vi "SerialServer.vi"(5 "Stop Refnum":refnum<vi>, 6 "Local Port":u16=16505) -> (0 "error out":errorcluster, 3 "FPGA VI Reference Out":refnum<k20>)   [LabVIEW 2013]
panel:
  out "Baud Rate":i32(ring)=1 items=["9600"=1, "19200"=2, "38400"=4, "57600"=8, "115200"=16, "230400"=32, "460800"=64, "921600"=128]
  out "OverRunError":bool
  in  "Flush on Close":bool
  out "UART TX count":u64
  out "UART RX count":u64
  out "TCP Bytes Out":u64
  out "Elements in UART TX Queue":i32
  out "Elements in UART RX Queue":i32
  out "TCP Bytes In":u64
  out "connection ID":refnum<k5>
  out "Connected?":bool
  out "Stopped?":bool caption="BeenStopped?"
  out "Remote Address":string
  out "Remote Port":u16
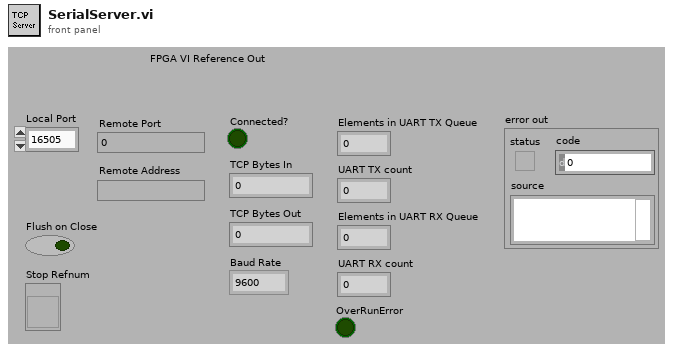
[diagram p1: front panel]
types:
  T1 = typedef "FPGA_Reference.ctl" = refnum<k20>
  T2 = enum16{"Standard", "Buffered", "CRLF", "Immediate"}
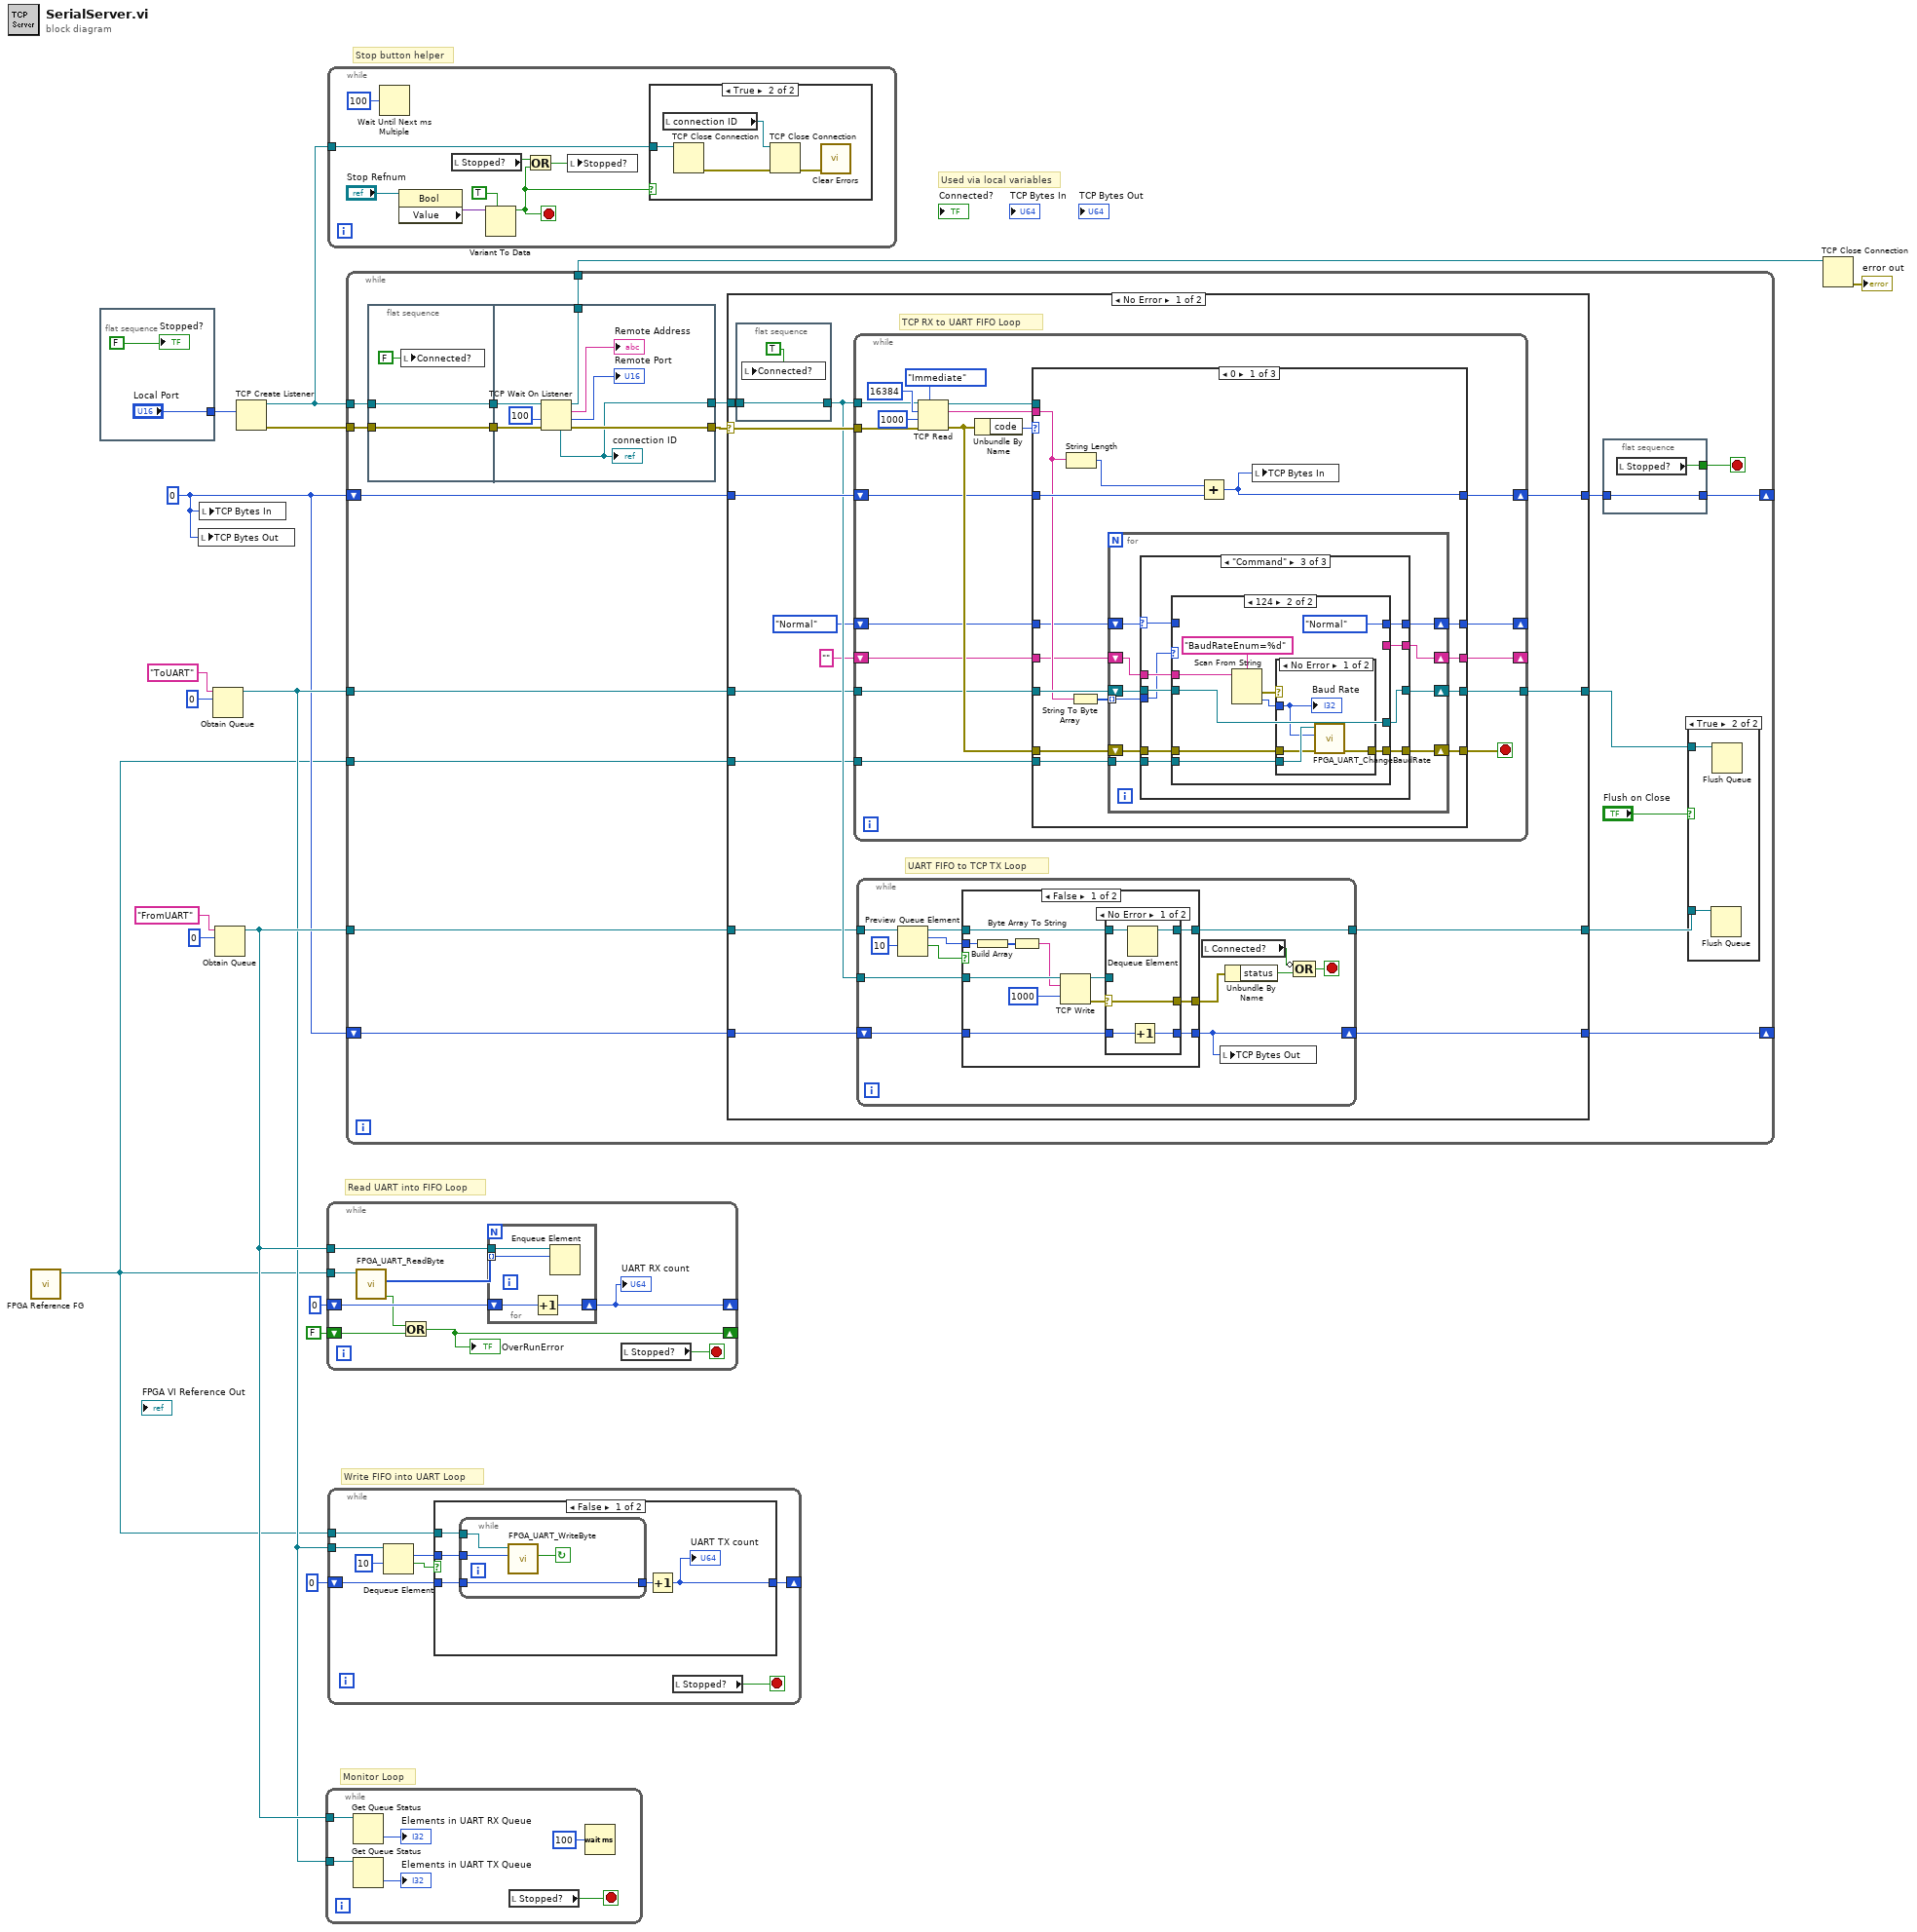
[diagram p0: block diagram]
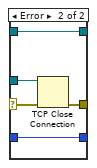
[diagram p5: hidden frame]
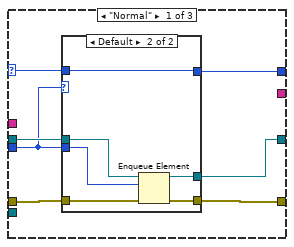
[diagram p7: hidden frame]
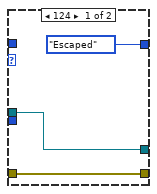
[diagram p8: hidden frame]
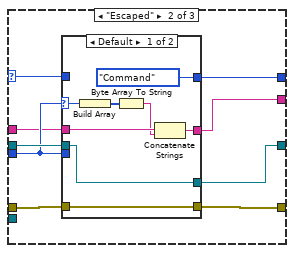
[diagram p9: hidden frame]
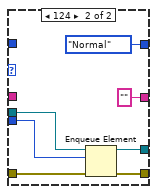
[diagram p10: hidden frame]
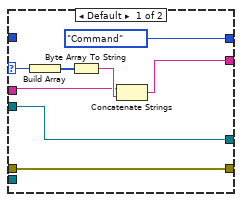
[diagram p11: hidden frame]
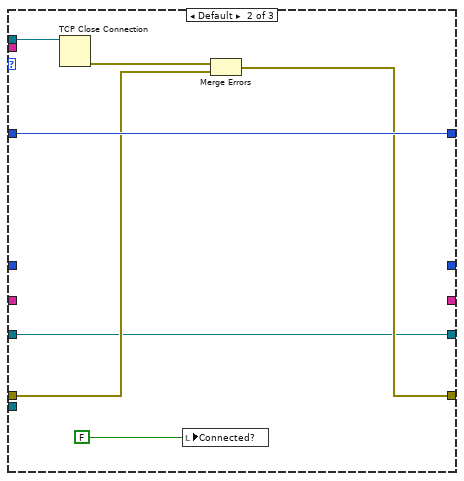
[diagram p13: hidden frame]
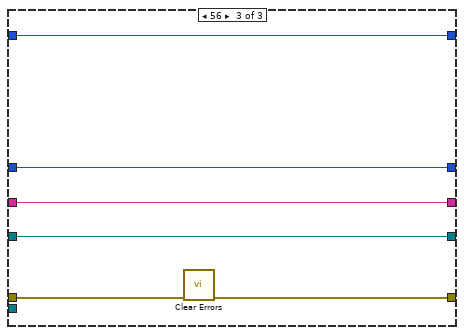
[diagram p14: hidden frame]
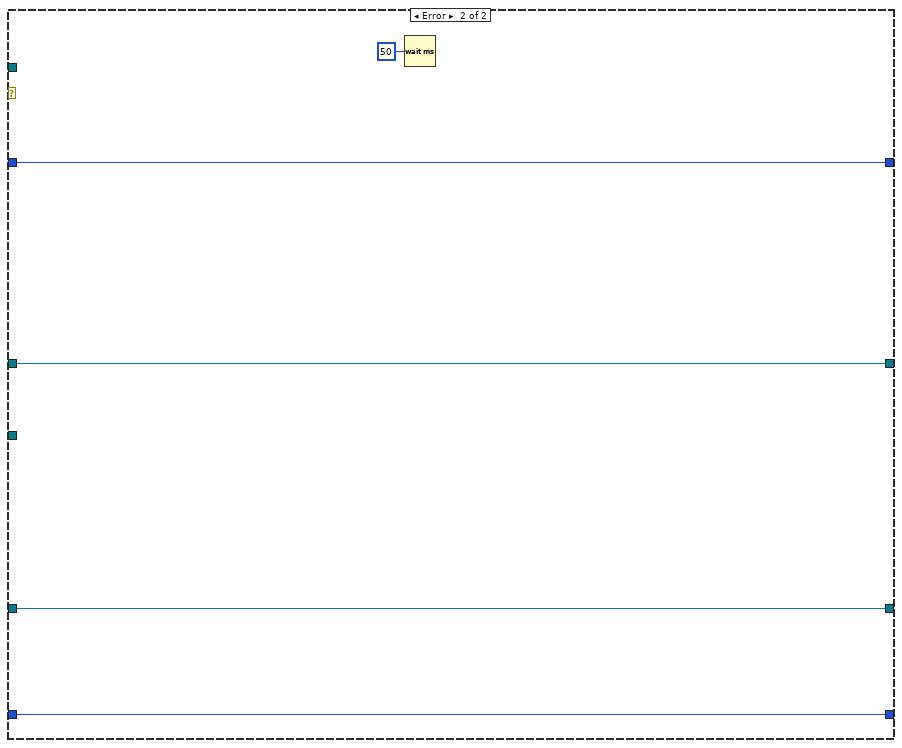
[diagram p15: hidden frame]
diagram:
  w8 = u64 0
  # "Monitor Loop"
  # "Write FIFO into UART Loop"
  # "Read UART into FIFO Loop"
  # "Stop button helper"
  # "Used via local variables"
  n1 = call "FPGA Reference FG.vi"() -> ("FPGA VI Reference Out"=w1:T1)  [unwired: 11 in]
  n2 = flat-sequence {
    tunnel: ["Local Port"] -> w3
    frame #0 {
      "Stopped?" <- FALSE ("Stopped?")
    }
  }
  n3 = local write "TCP Bytes Out"(w8) -> ()
  n4 = local write "TCP Bytes In"(w8) -> ()
  n5 = Obtain Queue(name (unnamed)="ToUART", element data type=u8 0) -> (queue out=w9:refnum<queue>)  [unwired: 3 in, 2 out]
  n6 = Obtain Queue(name (unnamed)="FromUART", element data type=u8 0) -> (queue out=w10:refnum<queue>)  [unwired: 3 in, 2 out]
  n7 = TCP Create Listener(10:w3) -> (0:w16:errorcluster, 3:w15:refnum<k5>)  [unwired: 1 in, 4 out]
  n8 = while {
    tunnel: w10 -> [w22]
    tunnel: w9 -> [w20]
    stop <- w24 stop-if-true
    n9 = Get Queue Status(queue=w22) -> (# elements in queue=→"Elements in UART RX Queue":i32)  [unwired: 1 in, 8 out]
    n10 = Get Queue Status(queue=w20) -> (# elements in queue=→"Elements in UART TX Queue":i32)  [unwired: 1 in, 8 out]
    n11 = local read "Stopped?"() -> (w24:bool)
    n12 = Wait (ms)(milliseconds to wait=u32 100) -> ()  [unwired: 1 out]
  }
  n13 = while {
    tunnel: w10 -> [w32]
    shift-right: [w30] -> _
    shift-left: u64 0 -> [w31]
    tunnel: w1 -> [w25]
    shift-right: [w26] -> _
    shift-left: FALSE -> [w27]
    stop <- w33 stop-if-true
    n14 = call "FPGA_UART_ReadByte.vi"("FPGA VI Reference In"=w25) -> ("OverRunError"=w28:bool, "Bytes"=w29:u8[])  [unwired: 9 out]
    n15 = Or(x=w28, y=w27) -> (x .or. y?=w26:bool)
    "OverRunError" <- w26
    n16 = for {
      tunnel: w32 -> [w37]
      tunnel: w29 -> [w34] mode=indexing
      shift-right: [w35] -> w30
      shift-left: w31 -> [w36]
      n17 = Increment(x=w36) -> (x+1=w35:u64)
      n18 = Enqueue Element(queue=w37, element=w34) -> ()  [unwired: 1 in, 4 out]
    }
    "UART RX count" <- w30
    n19 = local read "Stopped?"() -> (w33:bool)
  }
  n20 = while {
    tunnel: w15 -> [w44]
    stop <- w38 stop-if-true
    n21 = Wait Until Next ms Multiple(millisecond multiple=u32 100) -> ()  [unwired: 1 out]
    n22 = property class="Bool"(reference="Stop Refnum") -> ("Value"=w43:variant)  [unwired: 1 in, 2 out]
    n23 = local read "Stopped?"() -> (w39:bool)
    n24 = Variant To Data(type=TRUE ("stop"), Variant=w43) -> (data=w38:bool)  [unwired: 1 in, 1 out]
    n25 = Or(x=w39, y=w38) -> (x .or. y?=w40:bool)
    n26 = local write "Stopped?"(w40) -> ()
    n27 = case shown="True" w38 {
      tunnel: w44 -> [_ w46]
      frame False {
      }
      frame True {
        n28 = local read "connection ID"() -> (w48:refnum<k5>)
        n29 = TCP Close Connection(connection ID=w46) -> (error out=w47:errorcluster)  [unwired: 1 in, 2 out]
        n30 = TCP Close Connection(connection ID=w48, error in (no error)=w47) -> (error out=w49:errorcluster)  [unwired: 2 out]
        n31 = call <vilib>:"Clear Errors.vi"("error in (no error)"=w49) -> ()  [unwired: 7 out]
      }
    }
  }
  n32 = while {
    tunnel: w9 -> [w57]
    shift-right: [w51] -> _
    shift-left: u64 0 -> [w52]
    tunnel: w1 -> [w50]
    stop <- w53 stop-if-true
    n33 = Dequeue Element(queue=w57, timeout in ms (-1)=10) -> (element=w54:u8, timed out?=w55:bool)  [unwired: 1 in, 2 out]
    n34 = case shown="False" w55 {
      tunnel: w54 -> [w62 _]
      tunnel: w52 -> [w61 w67]
      tunnel: [w59 w67] -> w51
      tunnel: w50 -> [w58 _]
      frame False {
        n35 = while {
          tunnel: w62 -> [w65]
          tunnel: w61 -> [w66]
          tunnel: [w66] -> w60
          tunnel: w58 -> [w63]
          stop <- w64 continue-if-true
          n36 = call "FPGA_UART_WriteByte.vi"("Byte Value"=w65, "FPGA VI Reference In"=w63) -> ("Overflow?"=w64:bool)  [unwired: 2 in, 6 out]
        }
        n37 = Increment(x=w60) -> (x+1=w59:u64)
        "UART TX count" <- w59
      }
      frame True {
      }
    }
    n38 = local read "Stopped?"() -> (w53:bool)
  }
  n39 = while {
    tunnel: w15 -> [w85]
    tunnel: w16 -> [w86]
    shift-right: [w79] -> _
    shift-left: w8 -> [w81]
    tunnel: w9 -> [w78]
    tunnel: w10 -> [w75]
    shift-right: [w73] -> _
    shift-left: w8 -> [w74]
    tunnel: [w69] -> w5
    tunnel: w1 -> [w68]
    stop <- w82 stop-if-true
    n40 = flat-sequence {
      tunnel: w85 -> [w90]
      tunnel: w86 -> [w91]
      tunnel: [w91] -> w77
      tunnel: [w90] -> w76
      tunnel: w77 -> [w97]
      tunnel: w76 -> [w96]
      tunnel: [w95] -> w84
      tunnel: [w92] -> w83
      tunnel: [w93] -> w69
      frame #0 {
        n41 = local write "Connected?"(FALSE ("Connected?")) -> ()
      }
      frame #1 {
        n42 = TCP Wait On Listener(8:w97, 9:100 ("timeout ms (wait forever: -1)"), 11:w96) -> (0:w95:errorcluster, 1:→"Remote Port":u16, 2:→"Remote Address":string, 3:w93:refnum<k5>, 4:w92:refnum<k5>)  [unwired: 1 in]
        "connection ID" <- w92
      }
    }
    n43 = case shown="No Error" w84 {
      selector: w84 -> [w113 _]
      tunnel: w83 -> [w112 _]
      tunnel: w81 -> [w115 w287]
      tunnel: [w114 w287] -> w80
      tunnel: w78 -> [w107 w284]
      tunnel: w75 -> [w108 w285]
      tunnel: w74 -> [w110 w286]
      tunnel: [w109 w286] -> w73
      tunnel: [w106 w284] -> w72
      tunnel: [w105 w285] -> w71
      tunnel: w68 -> [w103 _]
      frame No Error {
        # "UART FIFO to TCP TX Loop"
        # "TCP RX to UART FIFO Loop"
        n44 = flat-sequence {
          tunnel: w112 -> [w153]
          tunnel: [w153] -> w111
          frame #0 {
            n45 = local write "Connected?"(TRUE ("Connected?")) -> ()
          }
        }
        n46 = while {
          tunnel: w113 -> [w166]
          shift-right: [w163] -> w114
          shift-left: w115 -> [w164]
          tunnel: w107 -> [w162]
          tunnel: w111 -> [w161]
          tunnel: [w160] -> w106
          shift-right: [w155] -> _
          shift-left: "" -> [w159]
          shift-right: [w156] -> _
          shift-left: enum16{"Normal", "Escaped", "Command"}."Normal" -> [w158]
          tunnel: w103 -> [w157]
          stop <- w167 stop-if-true
          n47 = TCP Read(connection ID=w161, bytes to read=16384, error in (no error)=w166, 7:T2."Immediate" ("mode (standard)"), 9:1000 ("timeout ms (25000)")) -> (connection ID out=w169:refnum<k5>, data out=w168:string, error out=w170:errorcluster)
          n48 = Unbundle By Name(w170) -> ("code"=w171:i32)
          n49 = case shown="0" w171 {
            tunnel: w170 -> [w181 w274 w282]
            tunnel: w169 -> [_ w275 _]
            tunnel: w168 -> [w183 _ _]
            tunnel: [w180 w272 w281] -> w167
            tunnel: w164 -> [w187 w276 w280]
            tunnel: [w186 w276 w280] -> w163
            tunnel: w162 -> [w185 w270 w279]
            tunnel: [w179 w270 w279] -> w160
            tunnel: w159 -> [w178 _ w277]
            tunnel: w158 -> [w177 _ w278]
            tunnel: w157 -> [w176 _ _]
            tunnel: [w175 _ w278] -> w156
            tunnel: [w174 _ w277] -> w155
            frame 0 {
              n50 = String Length(string=w183) -> (length=w184:i32)
              n51 = String To Byte Array(string=w183) -> (unsigned byte array=w182:u8[])
              n52 = for {
                tunnel: w182 -> [w193] mode=indexing
                shift-right: [w195] -> w180
                shift-left: w181 -> [w196]
                shift-right: [w194] -> w179
                shift-left: w185 -> [w197]
                shift-right: [w188] -> w174
                shift-left: w178 -> [w190]
                shift-right: [w191] -> w175
                shift-left: w177 -> [w192]
                tunnel: w176 -> [w189]
                n53 = case shown="\"Command\"" w192 {
                  selector: w192 -> [w198 w216 w242]
                  tunnel: w197 -> [w204 w222 w247]
                  tunnel: w193 -> [w200 w218 w239]
                  tunnel: w196 -> [w203 w221 w246]
                  tunnel: [w202 w220 w245] -> w195
                  tunnel: [w201 w219 w244] -> w194
                  tunnel: [w199 w217 w243] -> w191
                  tunnel: w190 -> [_ w215 w241]
                  tunnel: w189 -> [_ _ w240]
                  tunnel: [_ w214 w238] -> w188
                  frame "Normal" {
                    n54 = case shown="Default" w200 {
                      tunnel: w204 -> [w206 w213]
                      tunnel: w200 -> [_ w212]
                      tunnel: w203 -> [w205 w211]
                      tunnel: [w205 w210] -> w202
                      tunnel: [w206 w209] -> w201
                      tunnel: [enum16{"Normal", "Escaped", "Command"}."Escaped" w208] -> w199
                      tunnel: w198 -> [_ w208]
                      frame 124 {
                      }
                      frame Default {
                        n55 = Enqueue Element(queue=w213, element=w212, error in (no error)=w211) -> (queue out=w209:refnum<queue>, error out=w210:errorcluster)  [unwired: 2 out]
                      }
                    }
                  }
                  frame "Escaped" {
                    n56 = case shown="Default" w218 {
                      selector: w218 -> [w227 _]
                      tunnel: w222 -> [w229 w237]
                      tunnel: w218 -> [_ w236]
                      tunnel: w221 -> [w228 w235]
                      tunnel: [w228 w234] -> w220
                      tunnel: [w229 w233] -> w219
                      tunnel: [enum16{"Normal", "Escaped", "Command"}."Command" enum16{"Normal", "Escaped", "Command"}."Normal"] -> w217
                      tunnel: w216 -> [_ _]
                      tunnel: w215 -> [w225 _]
                      tunnel: [w223 ""] -> w214
                      frame Default {
                        n57 = Build Array(w227) -> (w226:u8[])
                        n58 = Byte Array To String(unsigned byte array=w226) -> (string=w224:string)
                        n59 = Concatenate Strings(w225, w224) -> (w223:string)
                      }
                      frame 124 {
                        n60 = Enqueue Element(queue=w237, element=w236, error in (no error)=w235) -> (queue out=w233:refnum<queue>, error out=w234:errorcluster)  [unwired: 2 out]
                      }
                    }
                  }
                  frame "Command" {
                    n61 = case shown="124" w239 {
                      selector: w239 -> [w252 _]
                      tunnel: w247 -> [w254 w263]
                      tunnel: w246 -> [w253 w258]
                      tunnel: [w253 w257] -> w245
                      tunnel: [w254 w263] -> w244
                      tunnel: [enum16{"Normal", "Escaped", "Command"}."Command" enum16{"Normal", "Escaped", "Command"}."Normal"] -> w243
                      tunnel: w242 -> [_ _]
                      tunnel: w241 -> [w249 w256]
                      tunnel: w240 -> [_ w259]
                      tunnel: [w248 _] -> w238
                      frame Default {
                        n62 = Build Array(w252) -> (w251:u8[])
                        n63 = Byte Array To String(unsigned byte array=w251) -> (string=w250:string)
                        n64 = Concatenate Strings(w249, w250) -> (w248:string)
                      }
                      frame 124 {
                        n65 = Scan From String(format string="BaudRateEnum=%d", input string=w256) -> (error out=w261:errorcluster, output 1=w260:i32)  [unwired: 3 in, 2 out]
                        n66 = case shown="No Error" w261 {
                          tunnel: w260 -> [w265 _]
                          tunnel: w259 -> [w268 _]
                          tunnel: w258 -> [w267 w269]
                          tunnel: [w266 w269] -> w257
                          frame No Error {
                            n67 = call "FPGA_UART_ChangeBaudRate.vi"("error  in"=w267, "Baud Rate Enum"=w265, "FPGA VI Reference In"=w268) -> ("error out"=w266:errorcluster)  [unwired: 6 in, 1 out]
                            "Baud Rate" <- w265
                          }
                          frame Error {
                          }
                        }
                      }
                    }
                  }
                }
              }
              n68 = Add(x=w184, y=w187) -> (x+y=w186:u64)
              n69 = local write "TCP Bytes In"(w186) -> ()
            }
            frame Default {
              n70 = TCP Close Connection(connection ID=w275) -> (error out=w273:errorcluster)  [unwired: 1 in, 2 out]
              n71 = local write "Connected?"(FALSE ("Connected?")) -> ()
              n72 = Merge Errors(w273, w274) -> (w272:errorcluster)
            }
            frame 56 {
              n73 = call <vilib>:"Clear Errors.vi"("error in (no error)"=w282) -> ("error out"=w281:errorcluster)  [unwired: 6 out]
            }
          }
        }
        n74 = while {
          tunnel: w111 -> [w124]
          tunnel: w108 -> [w127]
          tunnel: [w116] -> w105
          shift-right: [w120] -> w109
          shift-left: w110 -> [w122]
          stop <- w117 stop-if-true
          n75 = Preview Queue Element(queue=w127, timeout in ms (-1)=10) -> (queue out=w121:refnum<queue>, element=w125:u8, timed out?=w126:bool)  [unwired: 1 in, 1 out]
          n76 = case shown="False" w126 {
            tunnel: w125 -> [w139 _]
            tunnel: w124 -> [w140 _]
            tunnel: [w134 _] -> w123
            tunnel: w122 -> [w131 w152]
            tunnel: [w130 w152] -> w120
            tunnel: w121 -> [w132 w151]
            tunnel: [w129 w151] -> w116
            frame False {
              n77 = Build Array(w139) -> (w138:u8[])
              n78 = Byte Array To String(unsigned byte array=w138) -> (string=w137:string)
              n79 = TCP Write(connection ID=w140, data in=w137, 9:1000 ("timeout ms (25000)")) -> (connection ID out=w133:refnum<k5>, error out=w135:errorcluster)  [unwired: 1 in, 1 out]
              n80 = case shown="No Error" w135 {
                selector: w135 -> [w145 w149]
                tunnel: [w145 w148] -> w134
                tunnel: w133 -> [_ w150]
                tunnel: w132 -> [w144 w146]
                tunnel: w131 -> [w143 w147]
                tunnel: [w142 w147] -> w130
                tunnel: [w141 w146] -> w129
                frame No Error {
                  n81 = Dequeue Element(queue=w144) -> (queue out=w141:refnum<queue>)  [unwired: 2 in, 3 out]
                  n82 = Increment(x=w143) -> (x+1=w142:u64)
                }
                frame Error {
                  n83 = TCP Close Connection(connection ID=w150, error in (no error)=w149) -> (error out=w148:errorcluster)  [unwired: 2 out]
                }
              }
            }
            frame True {
            }
          }
          n84 = local read "Connected?"() -> (w119:bool)
          n85 = local write "TCP Bytes Out"(w120) -> ()
          n86 = Unbundle By Name(w123) -> ("status"=w118:bool)
          n87 = Compound Arithmetic op=OR(invert w119, w118) -> (w117:bool)
        }
      }
      frame Error {
        n88 = Wait (ms)(milliseconds to wait=u32 50) -> ()  [unwired: 1 out]
      }
    }
    n89 = flat-sequence {
      tunnel: [w101] -> w82
      tunnel: w80 -> [w100]
      tunnel: [w100] -> w79
      frame #0 {
        n90 = local read "Stopped?"() -> (w101:bool)
      }
    }
    n91 = case shown="True" "Flush on Close" {
      tunnel: w72 -> [_ w88]
      tunnel: w71 -> [_ w87]
      frame False {
      }
      frame True {
        n92 = Flush Queue(queue=w87) -> ()  [unwired: 1 in, 3 out]
        n93 = Flush Queue(queue=w88) -> ()  [unwired: 1 in, 3 out]
      }
    }
  }
  n94 = TCP Close Connection(connection ID=w5) -> (error out=→"error out":errorcluster)  [unwired: 2 in, 1 out]
